vi "Test_030620.vi"() -> ()   [LabVIEW 2020]
uses:
  <vilib>/Analysis/3filter.llb/Filter Passband Type.ctl
  <vilib>/Analysis/2dsp.llb/Power Spectrum (DBL).vi
  <vilib>/Analysis/3filter.llb/Butterworth Filter (DBL).vi
  <vilib>/gmath/NI_Gmath.lvlib
  <vilib>/Analysis/NI_AALPro.lvlib
  <vilib>/Analysis/NI_AALBase.lvlib
panel:
  in  "order":i32=2
  out "Waveform Graph":dbl[](graph)
  in  "range split":i32
  out "max index":dbl
  out "max":dbl
  out "Power spectrum":cluster{"X":dbl, "Y":dbl}[](graph)
  in  "Ring":u16(ring) items=["1", "2", "3", "1*2", "1*3", "2*3", "1*2*3"]
  in  "noise":bool
  in  "frequency 3":dbl=10.0 format="%0.2p"
  in  "offset (deg) 3":dbl format="%0.2p"
  in  "amplitude 3":dbl=1.0 format="%0.2p"
  in  "frequency 2":dbl=10.0 format="%0.2p"
  in  "offset (deg) 2":dbl format="%0.2p"
  in  "amplitude 2":dbl=1.0 format="%0.2p"
  in  "frequency":dbl=10.0 format="%0.2p"
  in  "offset (deg)":dbl format="%0.2p"
  in  "amplitude":dbl=1.0 format="%0.2p"
  out "Signal":cluster{"X":dbl, "Y":dbl}[](graph)
  in  "stop":bool
  in  "Length of signal (sec)":dbl
  in  "sampling":i32
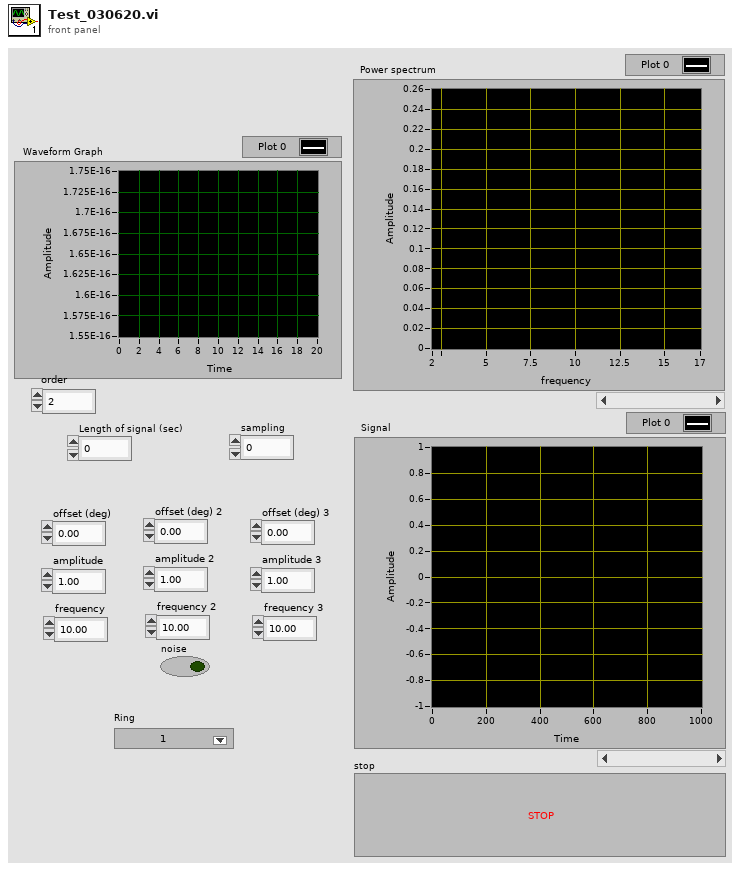
[diagram p1: front panel]
types:
  T1 = typedef "NI_AALBase.lvlib/Filter Passband Type.ctl" = enum32{"Lowpass", "Highpass", "Bandpass", "Bandstop"}
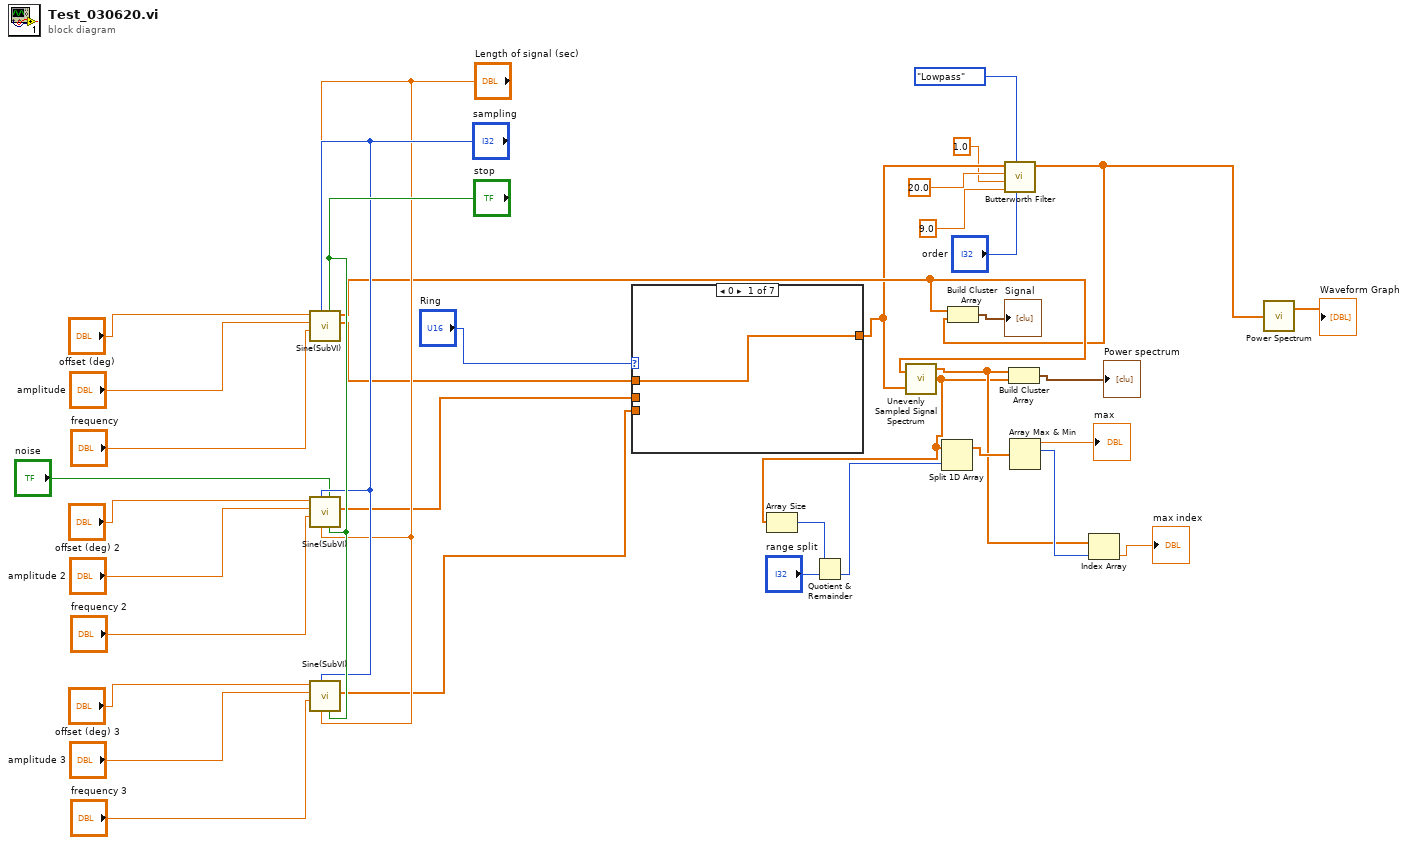
[diagram p0: block diagram]
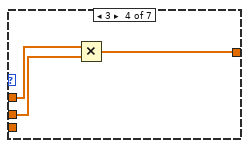
[diagram p4: hidden frame]
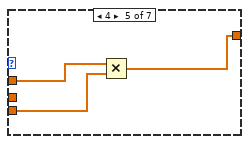
[diagram p5: hidden frame]
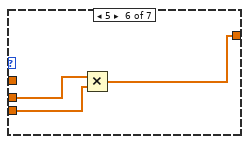
[diagram p6: hidden frame]
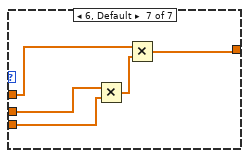
[diagram p7: hidden frame]
diagram:
  n1 = call "Sine(SubVI).vi"("stop"="stop", "length of signal"="Length of signal (sec)", "sampling"="sampling", "frequency"="frequency", "amplitude"="amplitude", "offset (deg)"="offset (deg)") -> ("amplitude"=w24:dbl[], "time"=w10:dbl[])  [unwired: 4 in]
  n2 = call "Sine(SubVI).vi"("stop"="stop", "error"="noise", "length of signal"="Length of signal (sec)", "sampling"="sampling", "frequency"="frequency 2", "amplitude"="amplitude 2", "offset (deg)"="offset (deg) 2") -> ("amplitude"=w23:dbl[])  [unwired: 3 in, 1 out]
  n3 = call "Sine(SubVI).vi"("stop"="stop", "length of signal"="Length of signal (sec)", "sampling"="sampling", "frequency"="frequency 3", "amplitude"="amplitude 3", "offset (deg)"="offset (deg) 3") -> ("amplitude"=w22:dbl[])  [unwired: 4 in, 1 out]
  n4 = case shown="0" "Ring" {
    tunnel: w24 -> [w38 _ _ w43 w46 _ w52]
    tunnel: [w38 w39 w40 w41 w44 w47 w50] -> w6
    tunnel: w23 -> [_ w39 _ w42 _ w49 w53]
    tunnel: w22 -> [_ _ w40 _ w45 w48 w54]
    frame 0 {
    }
    frame 1 {
    }
    frame 2 {
    }
    frame 3 {
      n5 = Multiply(x=w43, y=w42) -> (x*y=w41:dbl[])
    }
    frame 4 {
      n6 = Multiply(x=w46, y=w45) -> (x*y=w44:dbl[])
    }
    frame 5 {
      n7 = Multiply(x=w49, y=w48) -> (x*y=w47:dbl[])
    }
    frame 6, Default {
      n8 = Multiply(x=w53, y=w54) -> (x*y=w51:dbl[])
      n9 = Multiply(x=w52, y=w51) -> (x*y=w50:dbl[])
    }
  }
  n10 = call <vilib>:"Unevenly Sampled Signal Spectrum.vi"("XTime"=w10, "X"=w6) -> ("Power Spectrum FFT {X} Frequency"=w16:dbl[], "Power Spectrum FFT {X}"=w14:dbl[])  [unwired: 1 out]
  n11 = Array Size(array=w14) -> (size(s)=w12:i32)
  n12 = Quotient & Remainder(x=w12, y="range split") -> (floor(x/y)=w13:i32)  [unwired: 1 out]
  n13 = Split 1D Array(array=w14, index=w13) -> (first subarray=w18:dbl[])  [unwired: 1 out]
  n14 = call-poly <vilib>:"Butterworth Filter.vi"("order"="order", "filter type"=Filter_Passband_Type."Lowpass", "low cutoff freq: fl"=9.0, "high cutoff freq: fh"=1.0, "sampling freq: fs"=20.0, "X"=w6) -> ("Filtered X"=w4:dbl[])  [unwired: 2 in, 1 out]
  n15 = Build Cluster Array(w10, w4) -> (→"Signal":cluster{dbl, dbl}[])
  n16 = Build Cluster Array(w16, w14) -> (→"Power spectrum":cluster{dbl, dbl}[])
  n17 = Array Max & Min(array=w18) -> (max value=→"max":dbl, max index (indices)=w17:i32)  [unwired: 2 out]
  n18 = Index Array(array=w16, index=w17) -> (element=→"max index":dbl)
  n19 = call-poly <vilib>:"Power Spectrum.vi"("X"=w4) -> ("Power Spectrum"=→"Waveform Graph":dbl[])  [unwired: 1 out]
